vi "Clear All Values.vi"(8 "error in (no error)":errorcluster, 11 "Current Value Table":T1) -> (0 "error out":errorcluster, 3 "Current Value Table":T1)   [LabVIEW 2015, in "CurrentValueTable.lvlib" / "CurrentValueTable.lvclass"]
uses:
  CurrentValueTable.lvclass
  CurrentValueTable Reference.ctl
  CurrentValueTable.lvclass/CurrentValueTable.ctl
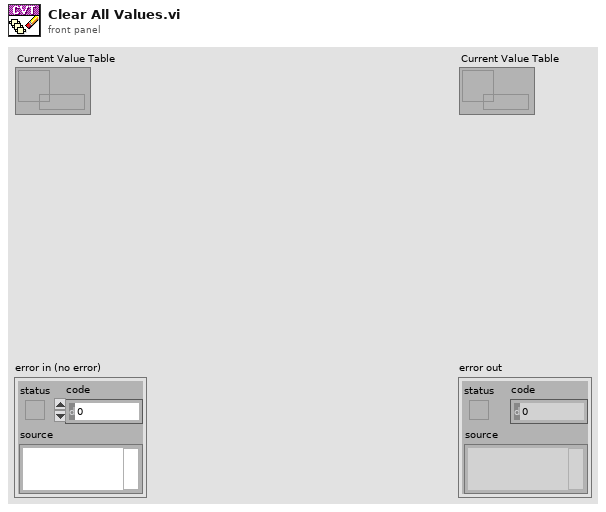
[diagram p1: front panel]
types:
  T1 = typedef "CurrentValueTable.lvlib/CurrentValueTable.lvclass/CurrentValueTable Reference.ctl" = refnum<data-value>
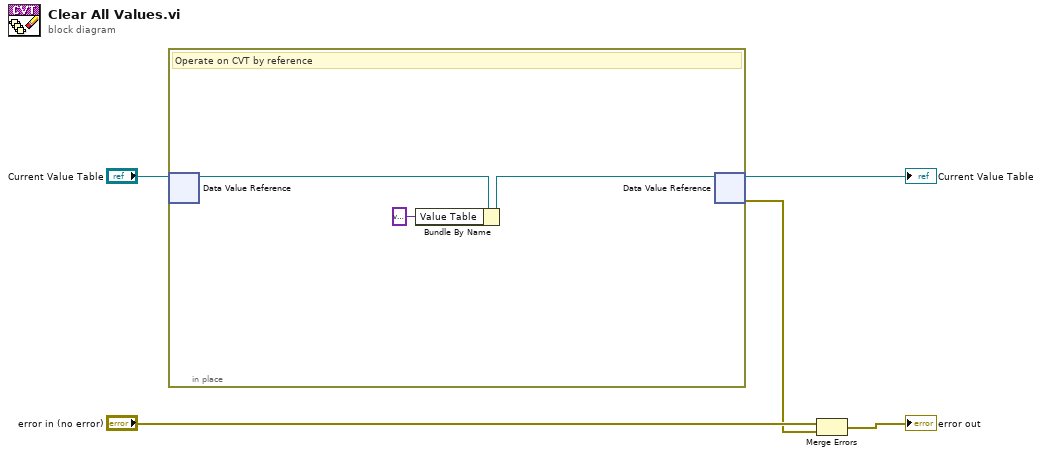
[diagram p0: block diagram]
diagram:
  n1 = in-place {
    # "Operate on CVT by reference"
    n2 = in-place-dvr #1("Current Value Table") -> (w8:refnum<class "CurrentValueTable.lvclass">)  [unwired: 1 out]
    n3 = Bundle By Name(cluster=w8, "Value Table"=variant) -> (w7:refnum<class "CurrentValueTable.lvclass">)
    n4 = in-place-dvr #1(w7) -> (→"Current Value Table":T1, w1:errorcluster)
  }
  n5 = Merge Errors("error in (no error)", w1) -> (→"error out":errorcluster)
